vi "respond to response.vi"(8 "error in (no error)":errorcluster caption="Fehler (Eingang, kein Fehler)", 10 "?":T1={"commandlist"="", "line"=0, "last response"="", "timeout"=0, "wait"=0, "erfolgreich"=FALSE, "next state"=enum."Start"}, 11 "Stoeraussendung Eingang":refnum<class "Stoeraussendung.lvclass"> caption="DNL_LabVIEW Object in") -> (0 "error out":errorcluster caption="Fehler (Ausgang)", 1 "read again?":bool, 2 "Cluster":T1={"commandlist"="", "line"=0, "last response"="", "timeout"=0, "wait"=0, "erfolgreich"=FALSE, "next state"=enum."Start"}, 3 "Stoeraussendung Ausgang":refnum<class "Stoeraussendung.lvclass"> caption="DNL_LabVIEW Object out")   [LabVIEW 2013, in "Stoeraussendung.lvclass"]
uses:
  Stoeraussendung.lvclass
  Main/controls/TestData.ctl
  Main/controls/TestStates.ctl
  TestInterface/TestInterface.lvclass
  lib/EMV-Test.lvlib
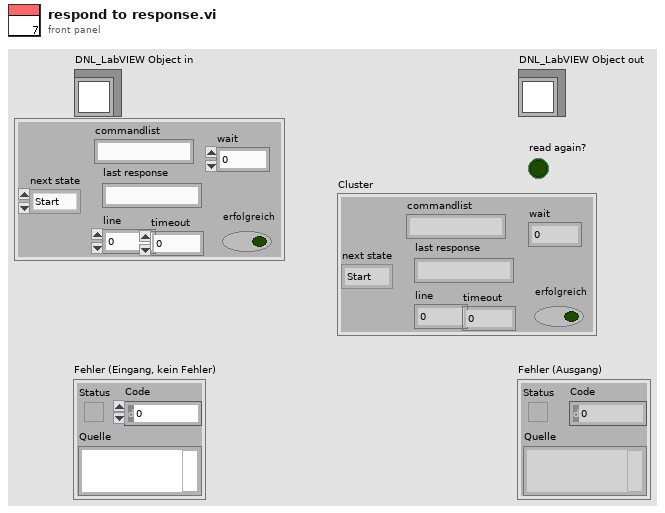
[diagram p1: front panel]
types:
  T1 = typedef "EMV-Test.lvlib/TestData.ctl" = cluster{"commandlist":string, "line":i32, "last response":string, "timeout":i32, "wait":u32, "erfolgreich":bool, "next state":T2}
  T2 = typedef "EMV-Test.lvlib/TestStates.ctl" = enum16{"check for pressed Buttons", "pause", "vorgefertigter Test", "manueller Test", "respond to response", "error", "Start", "Initialise", "open connection", "evaluate line", "wait for Response", "wait", "catch error", "close Connection", "end", "empty buffer"}
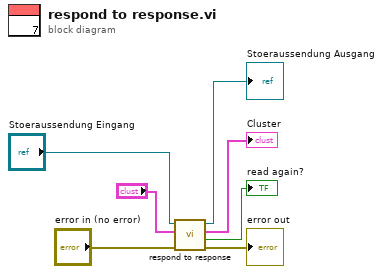
[diagram p0: block diagram]
diagram:
  n1 = call-parent "respond to response.vi"("error in (no error)"="error in (no error)", 10:"?", "TestInterface Eingang"="Stoeraussendung Eingang") -> ("error out"=→"error out":errorcluster, "read again?"=→"read again?":bool, "Cluster"=→"Cluster":T1, "TestInterface Ausgang"=→"Stoeraussendung Ausgang":refnum<class "Stoeraussendung.lvclass">)  [unwired: 5 in]
